vi "Update Elevator Call.vi"(8 "error in (no error)":errorcluster, 10 "Elevator Call":T1, 11 "Sim User Console Actor in":refnum<class "Sim User Console Actor.lvclass">) -> (0 "error out":errorcluster, 3 "Sim User Console Actor out":refnum<class "Sim User Console Actor.lvclass">)   [LabVIEW 2019]
uses:
  Elevator Controller/Elevator Controller Actor Messages/Wait for First Request Msg/Wait for First Request Msg.lvclass
  <vilib>/ActorFramework/Actor/Actor.lvclass
  Sim User Console Actor.lvclass
  C:/Workspace/CLA/Elevator AF 2nd/User Console Actor/User Console Actor/User Console Actor.lvclass
  C:/Program Files (x86)/National Instruments/LabVIEW 2019/vi.lib/ActorFramework/Actor/Actor.lvclass
  Elevator Call.ctl
panel:
  # "Fourth Floor"
  # "Third Floor"
  # "Second Floor"
  # "First Floor"
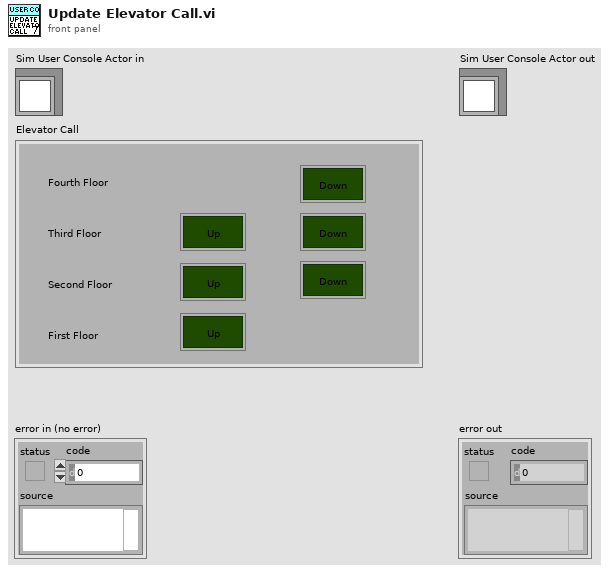
[diagram p1: front panel]
types:
  T1 = typedef "Simulated User Console Actor.lvlib/Sim User Console Actor.lvclass/Elevator Call.ctl" = cluster{"Up":bool, "Up 2":bool, "Up 3":bool, "Down":bool, "Down 2":bool, "Down 3":bool}
  T2 = typedef "Simulated User Console Actor.lvlib/Sim User Console Actor.lvclass/Floor Selection.ctl" = cluster{"Floor4":bool, "Floor 3":bool, "Floor2":bool, "Floor1":bool}
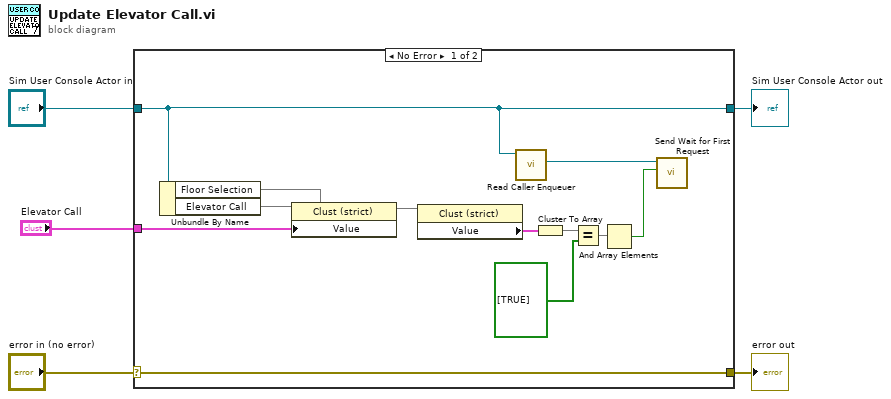
[diagram p0: block diagram]
diagram:
  n1 = case shown="No Error" "error in (no error)" {
    selector: "error in (no error)" -> [w16 w18]
    tunnel: [w16 w18] -> w4
    tunnel: [w13 w17] -> w2
    tunnel: "Sim User Console Actor in" -> [w13 w17]
    tunnel: "Elevator Call" -> [w14 _]
    frame No Error {
      n2 = Unbundle By Name(w13) -> ("Floor Selection"=w11, "Elevator Call"=w15)
      n3 = property class="Clust (strict)"(reference=w15, "Value"=w14) -> ()  [unwired: 1 in, 2 out]
      n4 = property class="Clust (strict)"(reference=w11) -> ("Value"=w10:T2)  [unwired: 1 in, 2 out]
      n5 = call <vilib>:"Read Caller Enqueuer.vi"("Actor"=w13) -> ("Caller Enqueuer"=w12:refnum<class "Message Enqueuer.lvclass">)  [unwired: 10 in]
      n6 = Cluster To Array(cluster=w10) -> (array=w9:bool[])
      n7 = Equal?(x=w9, y=bool[] [TRUE] ("array")) -> (x = y?=w7:bool[])
      n8 = And Array Elements(Boolean array=w7) -> (logical AND=w6:bool)
      n9 = call "Send Wait for First Request.vi"("be 1st floor?"=w6, "Message Enqueuer"=w12) -> ()  [unwired: 8 in, 2 out]
    }
    frame Error {
    }
  }
  "error out" <- w4
  "Sim User Console Actor out" <- w2
